vi "HV_Onstate_Multi.vi"(8 "On/Off":string[](array[string]), 11 "Channel":string[](array[string])) -> (3 "Output":string[](array[string]))   [LabVIEW 2018]
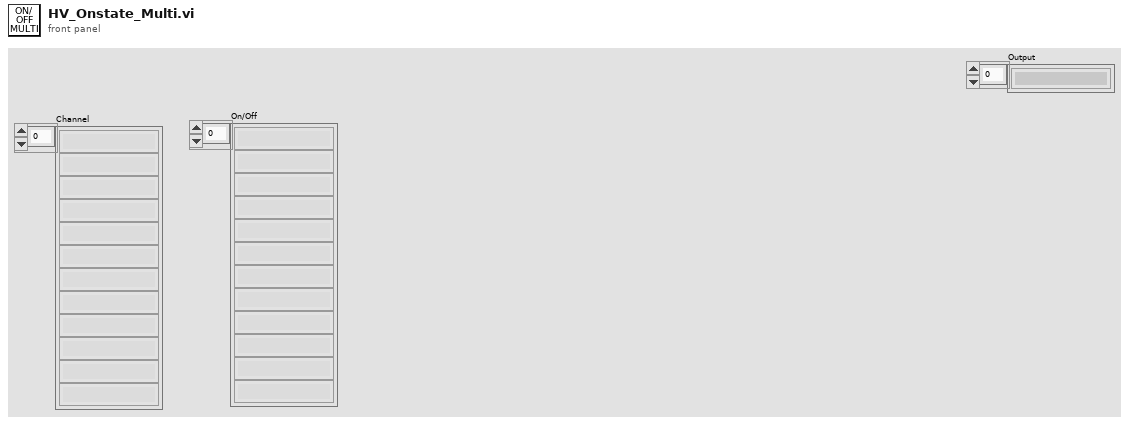
[diagram p1: front panel]
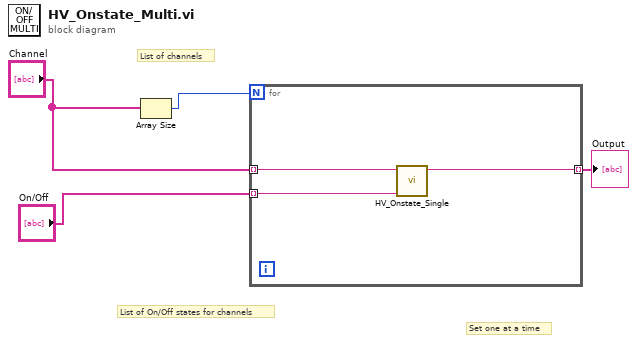
[diagram p0: block diagram]
diagram:
  # "Set one at a time"
  # "List of On/Off states for channels"
  # "List of channels"
  n1 = Array Size(array="Channel") -> (size(s)=w3:i32)
  n2 = for {
    N: w3 -> [_]
    tunnel: "Channel" -> [w7] mode=indexing
    tunnel: "On/Off" -> [w6] mode=indexing
    tunnel: [w5] -> w1 mode=indexing
    n3 = call "HV_Onstate_Single.vi"("On/Off"=w6, "Channel"=w7) -> ("standard output"=w5:string)  [unwired: 9 in]
  }
  "Output" <- w1
